vi "Stop Device.vi"(8 "error in":errorcluster, 11 "Alicat Device in":refnum<class "Alicat Device.lvclass">) -> (0 "error out":errorcluster, 3 "Alicat Device out":refnum<class "Alicat Device.lvclass">)   [LabVIEW 2014, in "Alicat Lib.lvlib" / "Alicat Device.lvclass"]
uses:
  Alicat Device.lvclass
  Alicat Device.lvclass/Alicat Device.ctl
  reusable/Session APIs/Serial/Serial Session.lvclass
  Configurable Device/Configurable Device.lvclass
  <userlib>/_Session Fwk/Session - Root.lvclass
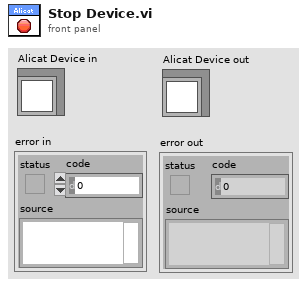
[diagram p1: front panel]
types:
  T1 = typedef "Serial Session.lvclass/Session Handle.ctl" = refnum<data-value>
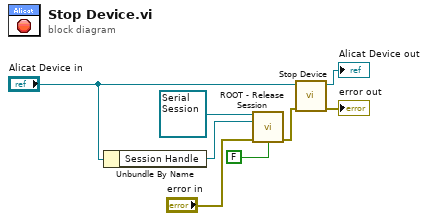
[diagram p0: block diagram]
diagram:
  n1 = Unbundle By Name("Alicat Device in") -> ("Session Handle"=w8:T1)
  n2 = call <userlib>:"ROOT - Release Session.vi"("OBJ - Session in"=refnum<class "Serial Session.lvclass"> refnum ("Serial Session"), "Session Handle in"=w8, "error in (no error)"="error in", "force destroy? (F)"=FALSE) -> ("error out"=w5:errorcluster)  [unwired: 10 in, 1 out]
  n3 = call-parent "Stop Device.vi"("error in"=w5, "Configurable Device in"="Alicat Device in") -> ("error out"=→"error out":errorcluster, "Configurable Device out"=→"Alicat Device out":refnum<class "Alicat Device.lvclass">)  [unwired: 8 in]
